vi "rotUk.vi"(8 "error in (no error)":errorcluster, 9 "uk Array":dbl[](array[numeric]), 10 "CamRot in":refnum<class "CamRot.lvclass">, 11 "ZTAAC in":refnum<class "ZTAAC.lvclass">) -> (0 "error out":errorcluster, 2 "Rotated uk Array":dbl[](array[numeric]), 3 "ZTAAC out":refnum<class "ZTAAC.lvclass">)   [LabVIEW 2016, in "OfcFunc.lvlib" / "ZTAAC.lvclass"]
doc: "Rotate uk based on the camera rotation angle."
uses:
  ZTAAC.lvclass
  CamRot/CamRot.lvclass
  StrictDef/DofGroup.ctl
  OfcFunc.lvlib
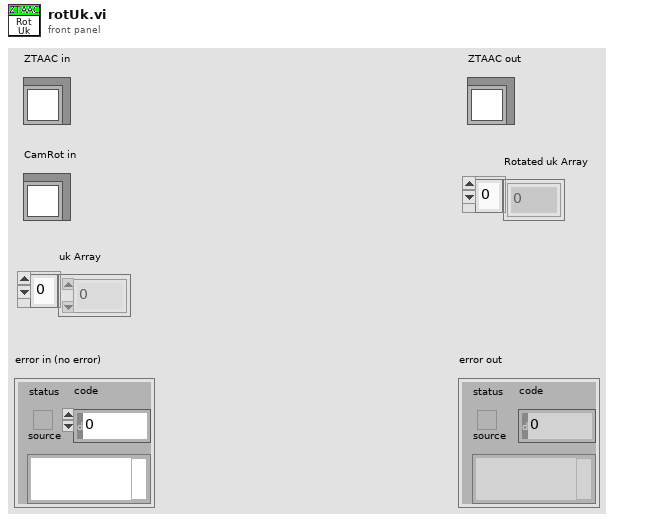
[diagram p1: front panel]
types:
  T1 = typedef "OfcFunc.lvlib/DofGroup.ctl" = enum16{"M2 Hex Pos", "Cam Hex Pos", "M1M3 Bend", "M2 Bend"}
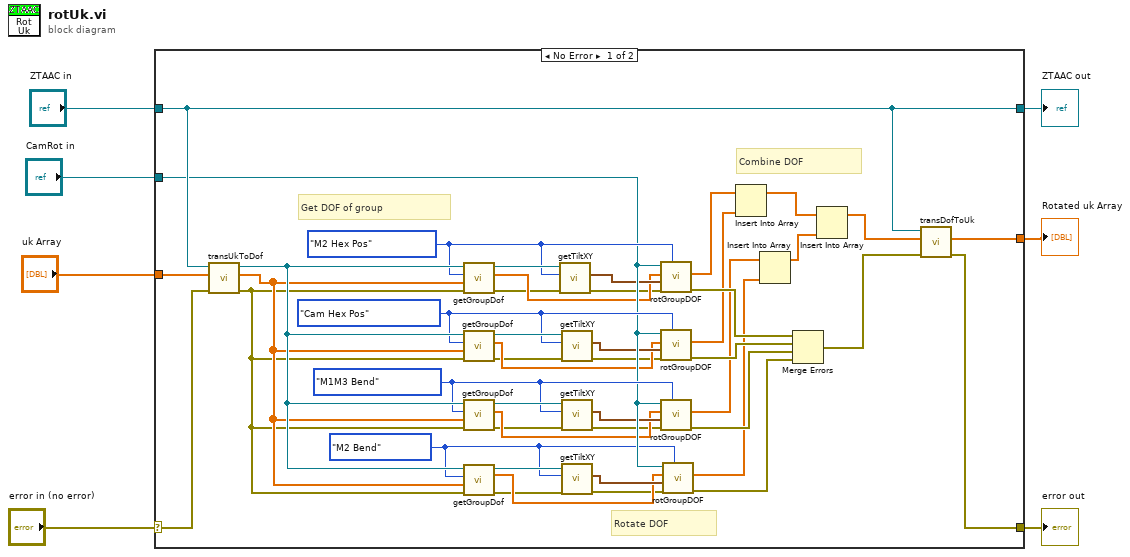
[diagram p0: block diagram]
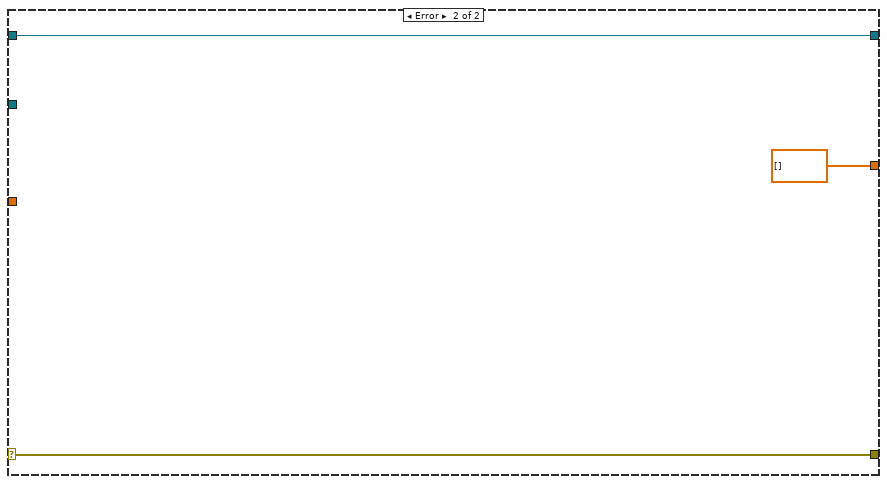
[diagram p2: hidden frame]
diagram:
  n1 = case shown="No Error" "error in (no error)" {
    selector: "error in (no error)" -> [w30 w55]
    tunnel: [w15 w55] -> w6
    tunnel: [w51 w54] -> w4
    tunnel: "ZTAAC in" -> [w51 w54]
    tunnel: "uk Array" -> [w52 _]
    tunnel: [w50 dbl[] [] ("uk Array")] -> w2
    tunnel: "CamRot in" -> [w40 _]
    frame No Error {
      w39 = DofGroup."M2 Bend" ("DOF Group")
      w41 = DofGroup."M1M3 Bend" ("DOF Group")
      w42 = DofGroup."Cam Hex Pos" ("DOF Group")
      w43 = DofGroup."M2 Hex Pos" ("DOF Group")
      # "Combine DOF"
      # "Rotate DOF"
      # "Get DOF of group"
      n2 = call "transUkToDof.vi"("error in (no error)"=w30, "uk Array"=w52, "ZTAAC in"=w51) -> ("error out"=w29:errorcluster, "State in DOF"=w48:dbl[], "ZTAAC out"=w49:refnum<class "ZTAAC.lvclass">)  [unwired: 6 in]
      n3 = call "getGroupDof.vi"("error in (no error)"=w29, "Input DOF"=w48, "DOF Group"=w43, "ZTAAC in"=w49) -> ("error out"=w28:errorcluster, "DOF"=w37:dbl[], "ZTAAC out"=w47:refnum<class "ZTAAC.lvclass">)  [unwired: 5 in]
      n4 = call "getGroupDof.vi"("error in (no error)"=w29, "Input DOF"=w48, "DOF Group"=w42, "ZTAAC in"=w49) -> ("error out"=w27:errorcluster, "DOF"=w35:dbl[], "ZTAAC out"=w46:refnum<class "ZTAAC.lvclass">)  [unwired: 5 in]
      n5 = call "getGroupDof.vi"("error in (no error)"=w29, "Input DOF"=w48, "DOF Group"=w41, "ZTAAC in"=w49) -> ("error out"=w26:errorcluster, "DOF"=w33:dbl[], "ZTAAC out"=w45:refnum<class "ZTAAC.lvclass">)  [unwired: 5 in]
      n6 = call "getGroupDof.vi"("error in (no error)"=w29, "Input DOF"=w48, "DOF Group"=w39, "ZTAAC in"=w49) -> ("error out"=w25:errorcluster, "DOF"=w31:dbl[], "ZTAAC out"=w44:refnum<class "ZTAAC.lvclass">)  [unwired: 5 in]
      n7 = call "getTiltXY.vi"("error in (no error)"=w28, "DOF Group"=w43, "ZTAAC in"=w47) -> ("error out"=w24:errorcluster, "Tilt Angle (arcsec)"=w38:cluster{"Tile X":dbl, "Tilt Y":dbl})  [unwired: 6 in, 1 out]
      n8 = call "getTiltXY.vi"("error in (no error)"=w27, "DOF Group"=w42, "ZTAAC in"=w46) -> ("error out"=w23:errorcluster, "Tilt Angle (arcsec)"=w36:cluster{"Tile X":dbl, "Tilt Y":dbl})  [unwired: 6 in, 1 out]
      n9 = call "getTiltXY.vi"("error in (no error)"=w26, "DOF Group"=w41, "ZTAAC in"=w45) -> ("error out"=w22:errorcluster, "Tilt Angle (arcsec)"=w34:cluster{"Tile X":dbl, "Tilt Y":dbl})  [unwired: 6 in, 1 out]
      n10 = call "getTiltXY.vi"("error in (no error)"=w25, "DOF Group"=w39, "ZTAAC in"=w44) -> ("error out"=w21:errorcluster, "Tilt Angle (arcsec)"=w32:cluster{"Tile X":dbl, "Tilt Y":dbl})  [unwired: 6 in, 1 out]
      n11 = call "rotGroupDOF.vi"("DOF Group"=w43, "error in (no error)"=w24, "Tilt Angle (arcsec)"=w38, "State in DOF"=w37, "CamRot in"=w40) -> ("error out"=w20:errorcluster, "Rotated State in DOF"=w14:dbl[])  [unwired: 4 in, 1 out]
      n12 = call "rotGroupDOF.vi"("DOF Group"=w42, "error in (no error)"=w23, "Tilt Angle (arcsec)"=w36, "State in DOF"=w35, "CamRot in"=w40) -> ("error out"=w19:errorcluster, "Rotated State in DOF"=w13:dbl[])  [unwired: 4 in, 1 out]
      n13 = call "rotGroupDOF.vi"("DOF Group"=w41, "error in (no error)"=w22, "Tilt Angle (arcsec)"=w34, "State in DOF"=w33, "CamRot in"=w40) -> ("error out"=w18:errorcluster, "Rotated State in DOF"=w12:dbl[])  [unwired: 4 in, 1 out]
      n14 = call "rotGroupDOF.vi"("DOF Group"=w39, "error in (no error)"=w21, "Tilt Angle (arcsec)"=w32, "State in DOF"=w31, "CamRot in"=w40) -> ("error out"=w17:errorcluster, "Rotated State in DOF"=w11:dbl[])  [unwired: 4 in, 1 out]
      n15 = Insert Into Array(array=w14, new element=w13) -> (w10:dbl[])  [unwired: 1 in]
      n16 = Insert Into Array(array=w12, new element=w11) -> (w9:dbl[])  [unwired: 1 in]
      n17 = Merge Errors(w20, w19, w18, w17) -> (w16:errorcluster)
      n18 = Insert Into Array(array=w10, new element=w9) -> (w8:dbl[])  [unwired: 1 in]
      n19 = call "transDofToUk.vi"("error in (no error)"=w16, "State in DOF"=w8, "ZTAAC in"=w51) -> ("error out"=w15:errorcluster, "uk Array"=w50:dbl[])  [unwired: 6 in, 1 out]
    }
    frame Error {
    }
  }
  "error out" <- w6
  "ZTAAC out" <- w4
  "Rotated uk Array" <- w2
